vi "Read Output.vi"(8 "error in (no error)":errorcluster, 11 "VISA resource name":refnum<visa-resource-name>) -> (0 "error out":errorcluster, 1 "Actual Current Level (A)":dbl format="%_5g", 2 "Actual Voltage Level (V)":dbl format="%_5g", 3 "VISA resource name out":refnum<visa-resource-name>)   [LabVIEW 2017, in "ADCMT 6240.lvlib"]
doc: "Returns the actual voltage level and actual current level."
uses:
  ADCMT 6240.lvlib
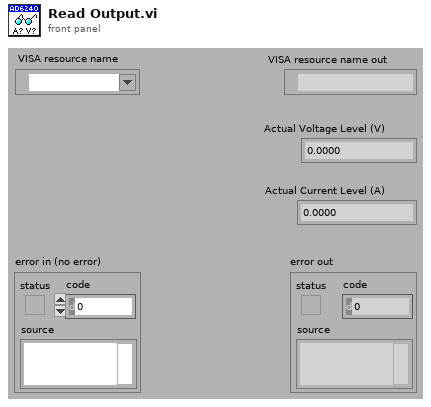
[diagram p1: front panel]
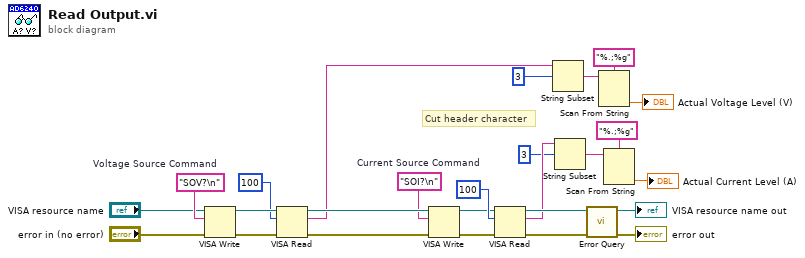
[diagram p0: block diagram]
diagram:
  w10 = "SOI?\n"  # Current Source Command
  w9 = "SOV?\n"  # Voltage Source Command
  # "Cut header character"
  n1 = VISA Write(VISA resource name="VISA resource name", write buffer=w9, error in (no error)="error in (no error)") -> (VISA resource name out=w25:refnum<visa-resource-name>, error out=w26:errorcluster)  [unwired: 1 out]
  n2 = VISA Read(VISA resource name=w25, byte count=u32 100, error in (no error)=w26) -> (VISA resource name out=w11:refnum<visa-resource-name>, read buffer=w1:string, error out=w12:errorcluster)  [unwired: 1 out]
  n3 = VISA Write(VISA resource name=w11, write buffer=w10, error in (no error)=w12) -> (VISA resource name out=w17:refnum<visa-resource-name>, error out=w16:errorcluster)  [unwired: 1 out]
  n4 = VISA Read(VISA resource name=w17, byte count=u32 100, error in (no error)=w16) -> (VISA resource name out=w14:refnum<visa-resource-name>, read buffer=w6:string, error out=w13:errorcluster)  [unwired: 1 out]
  n5 = String Subset(string=w1, offset (0)=3) -> (substring=w2:string)  [unwired: 1 in]
  n6 = String Subset(string=w6, offset (0)=3) -> (substring=w4:string)  [unwired: 1 in]
  n7 = call "Error Query.vi"("error in (no error)"=w13, "VISA resource name"=w14) -> ("error out"=→"error out":errorcluster, "VISA resource name out"=→"VISA resource name out":refnum<visa-resource-name>)  [unwired: 6 in, 2 out]
  n8 = Scan From String(format string="%.;%g", input string=w2) -> (output 1=→"Actual Voltage Level (V)":dbl)  [unwired: 3 in, 3 out]
  n9 = Scan From String(format string="%.;%g", input string=w4) -> (output 1=→"Actual Current Level (A)":dbl)  [unwired: 3 in, 3 out]
